vi "Transverse_Set.vi"   [LabVIEW 2019]
uses:
  Climb_Transverse_Control_States.ctl
  Globals/Climb_Globals.vi
types:
  T1 = typedef "Climb_Transverse_Control_States.ctl" = enum16{"No-Op", "Manual", "Auto-Balancing"}
  T2 = typedef "Climb_Transverse_Cluster.ctl" = cluster{"Auto-Balance?":bool, "Transverse_Throttle":dbl, "Control_States":T1}
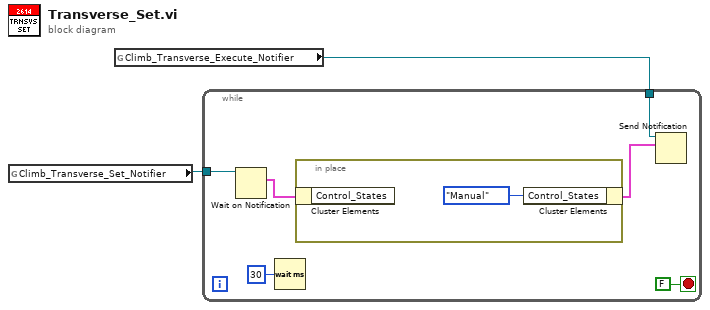
[diagram p0: block diagram]
diagram:
  n1 = global read "Climb_Globals.vi" "Climb_Transverse_Set_Notifier"() -> (w2:refnum<notifier>)
  n2 = global read "Climb_Globals.vi" "Climb_Transverse_Execute_Notifier"() -> (w1:refnum<notifier>)
  n3 = while {
    tunnel: w2 -> [w7]
    tunnel: w1 -> [w4]
    stop <- FALSE stop-if-true
    n4 = Wait on Notification(notifier=w7) -> (notification=w6:T2)  [unwired: 3 in, 3 out]
    n5 = Wait (ms)(milliseconds to wait=u32 30) -> ()  [unwired: 1 out]
    n6 = in-place {
      n7 = in-place-cluster #1(w6) -> ()  [unwired: 1 out]
      n8 = in-place-cluster #1("Control_States"=Climb_Transverse_Control_States."Manual") -> (w5:T2)
    }
    n9 = Send Notification(notification=w5, notifier=w4) -> ()  [unwired: 1 in, 2 out]
  }
